vi "AprilTag position on field.vi"(10 "AprilTag Number":i32=68) -> (2 "Target height to center (in)":dbl)   [LabVIEW 2025]
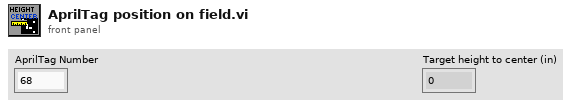
[diagram p1: front panel]
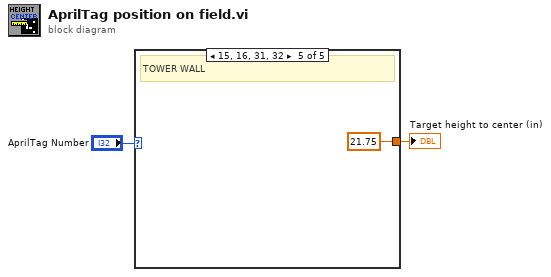
[diagram p0: block diagram]
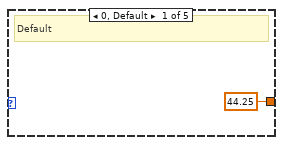
[diagram p2: hidden frame]
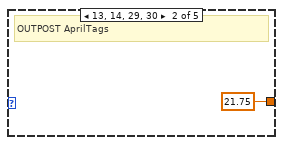
[diagram p3: hidden frame]
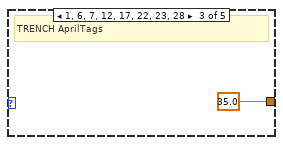
[diagram p4: hidden frame]
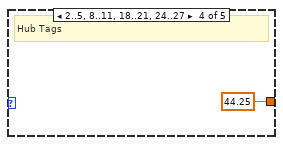
[diagram p5: hidden frame]
diagram:
  n1 = case shown="15, 16, 31, 32" "AprilTag Number" {
    tunnel: [44.25 21.75 35.0 44.25 21.75] -> w1
    frame 0, Default {
      # "Default"
    }
    frame 13, 14, 29, 30 {
      # "OUTPOST AprilTags"
    }
    frame 1, 6, 7, 12, 17, 22, 23, 28 {
      # "TRENCH AprilTags"
    }
    frame 2..5, 8..11, 18..21, 24..27 {
      # "Hub Tags"
    }
    frame 15, 16, 31, 32 {
      # "TOWER WALL"
    }
  }
  "Target height to center (in)" <- w1
